vi "Project VI.vi"() -> ()   [LabVIEW 2022 SP3]
uses:
  <vilib>/MakerHub/LINX/Public/Peripherals/Digital/Digital Write 1 Chan.vi
  <vilib>/MakerHub/LINX/Public/Peripherals/Digital/Digital Read 1 Chan.vi
  <vilib>/MakerHub/LINX/Public/Peripherals/Digital/Digital Write N Chans.vi
  <vilib>/MakerHub/LINX/Public/Peripherals/Digital/Digital Read N Chans.vi
  <vilib>/MakerHub/LINX/Private/Local IO/LinxDigitalWrite.vi
  <vilib>/MakerHub/LINX/Public/Utilities/Check Channel.vi
  <vilib>/MakerHub/LINX/Private/Local IO/LinxDigitalRead.vi
  <vilib>/MakerHub/LINX/Public/Utilities/Open Serial.vi
  <vilib>/MakerHub/LINX/Public/Sensors/Temperature/TMP3x/TMP35.vi
  <vilib>/MakerHub/LINX/Private/Utilties/Generate Error.vi
  <vilib>/MakerHub/LINX/LMH-LINX.lvlib
  <vilib>/MakerHub/LINX/Public/Sensors/Temperature/TMP3x/TMP3x.lvlib
panel:
  out "Light on/off":bool
  out "Buzzer":bool
  out "Motion":bool
  in  "Error In":errorcluster
  out "MODERATE":bool
  out "COLD":bool
  out "HOT":bool
  out "Temperature Chart":dbl(graph)
  in  "Minimum":dbl(slide) scale=0.0..50.0
  in  "Maximum":dbl(slide) scale=0.0..50.0
  out "Error Out":errorcluster
  in  "STOP":bool
  out "Loop Rate (Hz)":u32
  in  "Analog Channel":u8
  out "Thermometer":dbl(slide) scale=0.0..100.0
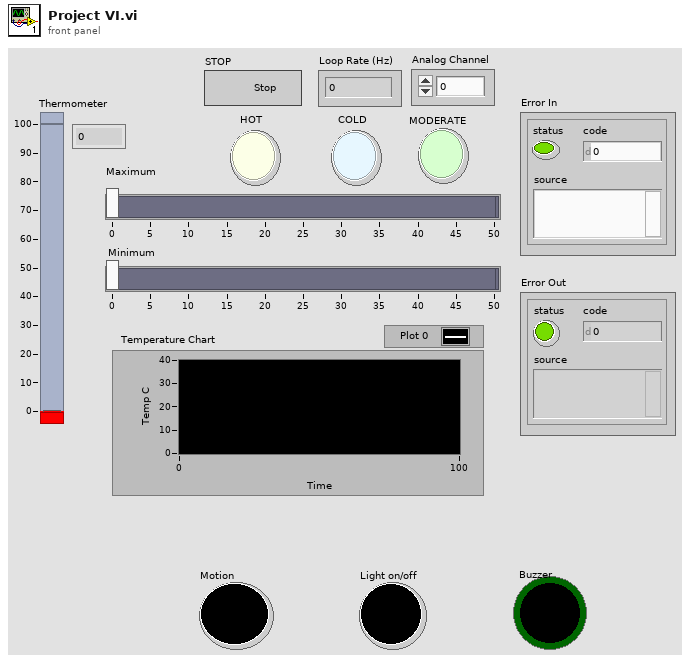
[diagram p1: front panel]
types:
  T1 = typedef "LMH-LINX.lvlib/LINX Ref.ctl" = cluster{"IO":T2, "Interface":T3, "LINX Device Config":T4}
  T2 = typedef "LMH-LINX.lvlib/Platform.ctl" = enum16{"Remote", "Local"}
  T3 = typedef "LMH-LINX.lvlib/Interface.ctl" = enum16{"Serial", "TCP"}
  T4 = typedef "LMH-LINX.lvlib/Device.lvlib/LINX Device Config.ctl" = cluster{"Interface":T3, "COM Port":refnum<visa-resource-name>, "TCP Configuration":T5, "Device Family":u8, "Device ID":u8, "Device Name":string, "TCP Ref":refnum<k5>, "Channels":T6}
  T5 = typedef "LMH-LINX.lvlib/Device.lvlib/TCP Config.ctl" = cluster{"IP Address":string, "Port":u16}
  T6 = typedef "LMH-LINX.lvlib/Channels.ctl" = cluster{"DI":u8[], "DO":u8[], "AI":u8[], "AO":u8[], "PWM":u8[], "QE":u8[], "UART":u8[], "I2C 2":u8[], "SPI":u8[], "CAN":u8[], "Servo":u8[], "AI Ref (V)":dbl, "AI Resolution (Bits)":u8, "AO Ref (V)":dbl, "AO Resolution (Bits)":u8}
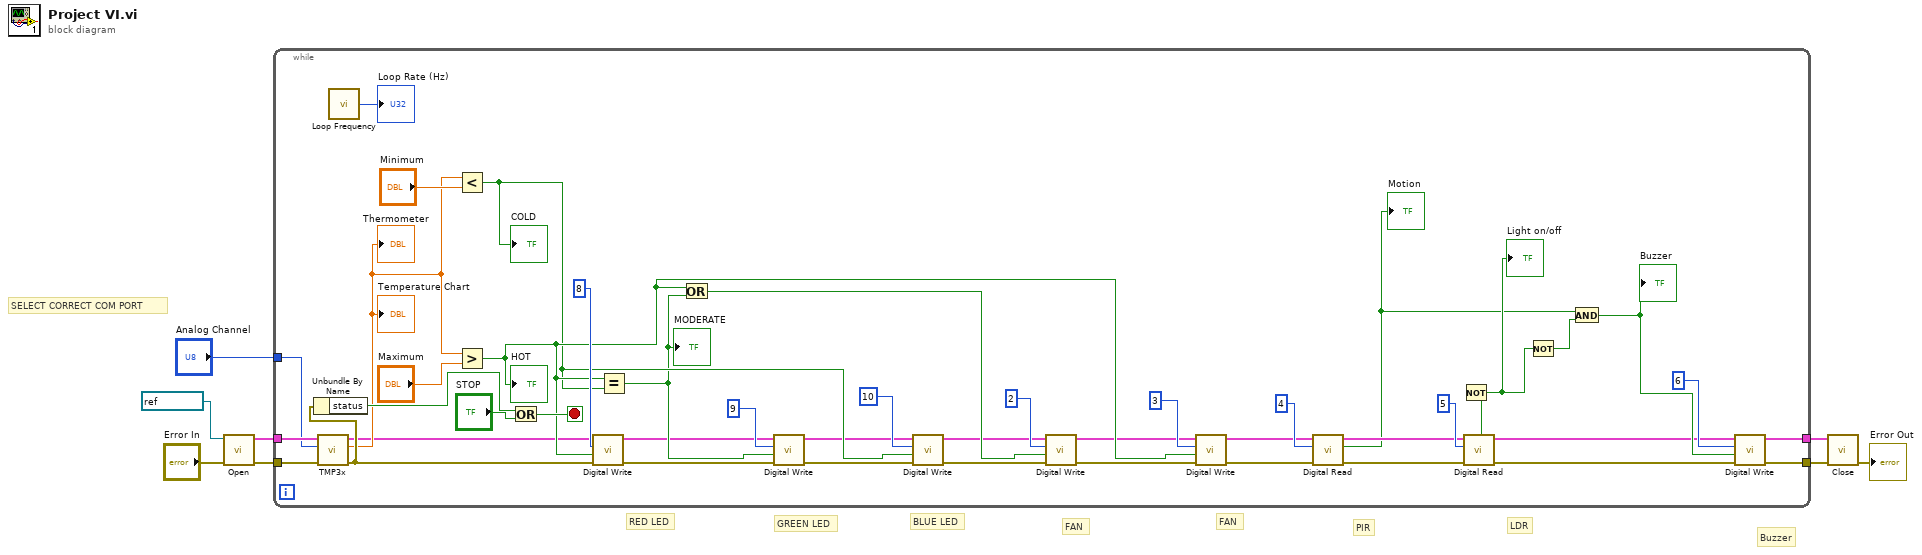
[diagram p0: block diagram]
diagram:
  # "Buzzer"
  # "LDR"
  # "PIR"
  # "FAN"
  # "SELECT CORRECT COM PORT"
  # "FAN"
  # "BLUE LED"
  # "GREEN LED"
  # "RED LED"
  n1 = call-poly <vilib>:"Open.vi"("Error In"="Error In", "Serial Port"=refnum<visa-resource-name> "COM8") -> ("Error Out"=w7:errorcluster, "LINX Resource"=w8:T1)  [unwired: 7 in, 1 out]
  n2 = while {
    tunnel: w8 -> [w53]
    tunnel: w7 -> [w52]
    tunnel: "Analog Channel" -> [w51]
    tunnel: [w28] -> w2
    tunnel: [w27] -> w1
    stop <- w47 stop-if-true
    n3 = call-poly <vilib>:"TMP3x.vi"("Error In"=w52, "Analog Channel"=w51, "LINX Resource"=w53) -> ("Error Out"=w44:errorcluster, "Temp C"=w38:dbl, "LINX Resource"=w17:T1)  [unwired: 6 in]
    "Thermometer" <- w38
    "Temperature Chart" <- w38
    n4 = Unbundle By Name(w44) -> ("status"=w48:bool)
    n5 = call <vilib>:"Loop Frequency.vi"() -> ("Loop Rate (Hz)"=→"Loop Rate (Hz)":u32)
    n6 = Less?(x=w38, y="Minimum") -> (x < y?=w21:bool)
    "COLD" <- w21
    n7 = Greater?(x=w38, y="Maximum") -> (0:w33:bool)
    "HOT" <- w33
    n8 = Or(x=w48, y="STOP") -> (x .or. y?=w47:bool)
    n9 = call-poly <vilib>:"Digital Write.vi"("Error In"=w44, "Output Value"=w33, "DO Channel"=u8 8, "LINX Resource"=w17) -> ("Error Out"=w45:errorcluster, "LINX Resource"=w16:T1)  [unwired: 6 in]
    n10 = Equal?(x=w33, y=w21) -> (x = y?=w20:bool)
    "MODERATE" <- w20
    n11 = Or(x=w33, y=w20) -> (x .or. y?=w32:bool)
    n12 = call-poly <vilib>:"Digital Write.vi"("Error In"=w45, "Output Value"=w20, "DO Channel"=u8 9, "LINX Resource"=w16) -> ("Error Out"=w46:errorcluster, "LINX Resource"=w15:T1)  [unwired: 6 in]
    n13 = call-poly <vilib>:"Digital Write.vi"("Error In"=w46, "Output Value"=w21, "DO Channel"=u8 10, "LINX Resource"=w15) -> ("Error Out"=w37:errorcluster, "LINX Resource"=w14:T1)  [unwired: 6 in]
    n14 = call-poly <vilib>:"Digital Write.vi"("Error In"=w37, "Output Value"=w32, "DO Channel"=u8 2, "LINX Resource"=w14) -> ("Error Out"=w35:errorcluster, "LINX Resource"=w13:T1)  [unwired: 6 in]
    n15 = call-poly <vilib>:"Digital Write.vi"("Error In"=w35, "Output Value"=w33, "DO Channel"=u8 3, "LINX Resource"=w13) -> ("Error Out"=w31:errorcluster, "LINX Resource"=w12:T1)  [unwired: 6 in]
    n16 = call-poly <vilib>:"Digital Read.vi"("Error In"=w31, "DI Channel"=u8 4, "LINX Resource"=w12) -> ("Error Out"=w30:errorcluster, "DI Value"=w10:bool, "LINX Resource"=w11:T1)  [unwired: 6 in]
    "Motion" <- w10
    n17 = call-poly <vilib>:"Digital Read.vi"("Error In"=w30, "DI Channel"=u8 5, "LINX Resource"=w11) -> ("Error Out"=w29:errorcluster, "DI Value"=w19:bool, "LINX Resource"=w9:T1)  [unwired: 6 in]
    n18 = Not(x=w19) -> (.not. x?=w18:bool)
    "Light on/off" <- w18
    n19 = Not(x=w18) -> (.not. x?=w23:bool)
    n20 = And(x=w10, y=w23) -> (x .and. y?=w22:bool)
    "Buzzer" <- w22
    n21 = call-poly <vilib>:"Digital Write.vi"("Error In"=w29, "Output Value"=w22, "DO Channel"=u8 6, "LINX Resource"=w9) -> ("Error Out"=w27:errorcluster, "LINX Resource"=w28:T1)  [unwired: 6 in]
  }
  n22 = call <vilib>:"Close.vi"("Error In"=w1, "LINX Resource"=w2) -> ("Error Out"=→"Error Out":errorcluster)  [unwired: 9 in]
